vi "Interface.vi"() -> ()   [LabVIEW 2020]
panel:
  out "rendering":refnum<vi>(3d-picture)
  in  "bucket angle":dbl
  in  "arm angle":dbl
  in  "boom angle":dbl
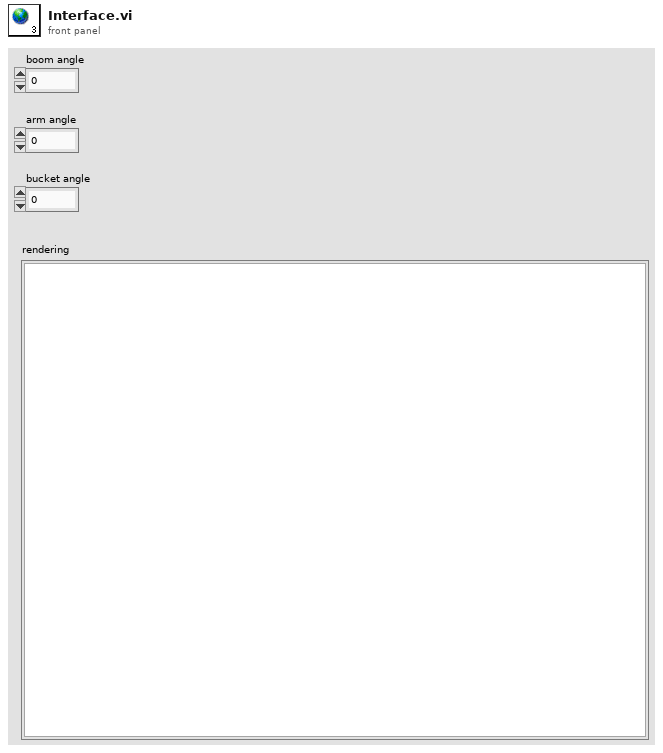
[diagram p1: front panel]
diagram:
